vi "Receive Value Change Event.vi"(8 "error in (no error)":errorcluster, 10 "ValueChangeMsg":refnum<class "ValueChangeMsg.lvclass">, 11 "IAttribute Data Type View In":refnum<class "IAttribute Data Type View.lvclass">) -> (0 "error out":errorcluster, 3 "IAttribute Data Type View Out":refnum<class "IAttribute Data Type View.lvclass">)   [LabVIEW 2017, in "IAttribute Data Type View.lvclass"]
doc: "<License>\nCopyright © 2017 Composed Systems, LLC | All rights reserved\nwww.composed.io\n\nAuthor: Ethan Stern <ethan.stern@composed.io>\n\nThis software is provided \"AS IS\" WITHOUT WARRANTIES, either express or implied, AND IS FOR EDUCATIONAL PURPOSES ONLY.\n</License>"
uses:
  IAttribute Data Type View.lvclass
  <vilib>/gpm_packages/@cs/mva-viewable/Source/ActorEvents/IEventAggregator Messages/ValueChangeMsg/ValueChangeMsg.lvclass
  <vilib>/ActorFramework/Actor/Actor.lvclass
  ITest Executive Builder Dialog Messages/Update Active Attribute Value Msg/Update Active Attribute Value Msg.lvclass
  C:/Program Files (x86)/National Instruments/LabVIEW 2017/vi.lib/ActorFramework/Actor/Actor.lvclass
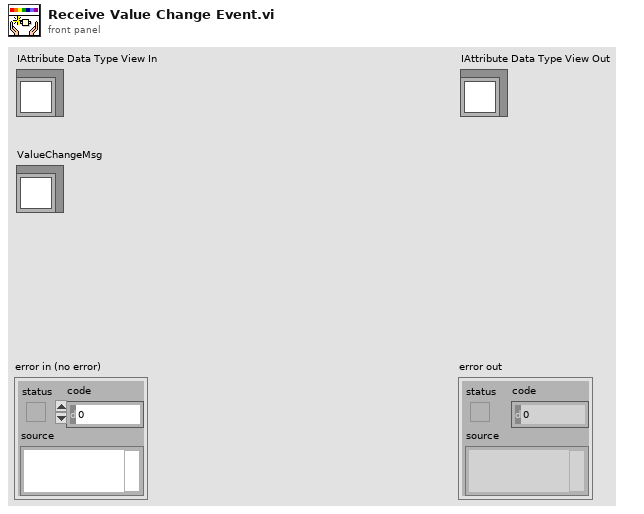
[diagram p1: front panel]
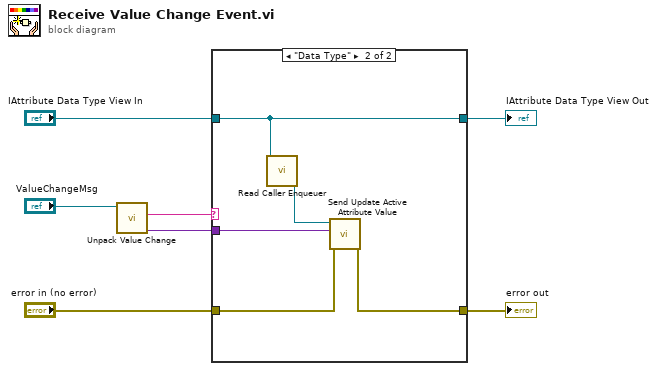
[diagram p0: block diagram]
diagram:
  n1 = call <vilib>:"Unpack Value Change.vi"("ValueChangeMsg"="ValueChangeMsg") -> ("New Value"=w1:variant, "Control Label"=w6:string)  [unwired: 6 in, 3 out]
  n2 = case shown="\"Data Type\"" w6 {
    tunnel: [w8 w14] -> w5
    tunnel: "IAttribute Data Type View In" -> [w8 w14]
    tunnel: [w9 w12] -> w3
    tunnel: "error in (no error)" -> [w9 w13]
    tunnel: w1 -> [_ w11]
    frame Default {
    }
    frame "Data Type" {
      n3 = call <vilib>:"Read Caller Enqueuer.vi"("Actor"=w14) -> ("Caller Enqueuer"=w10:refnum<class "Message Enqueuer.lvclass">)  [unwired: 10 in]
      n4 = call "Send Update Active Attribute Value.vi"("error in (no error)"=w13, "Data"=w11, "Message Enqueuer"=w10) -> ("error out"=w12:errorcluster)  [unwired: 7 in, 1 out]
    }
  }
  "error out" <- w3
  "IAttribute Data Type View Out" <- w5
